vi "test2.vi"() -> ()   [LabVIEW 2024]
panel:
  out "transmission time":dbl
  out "unsigned byte array":u8[](array[numeric])
  out "data out":string
  in  "stop":bool
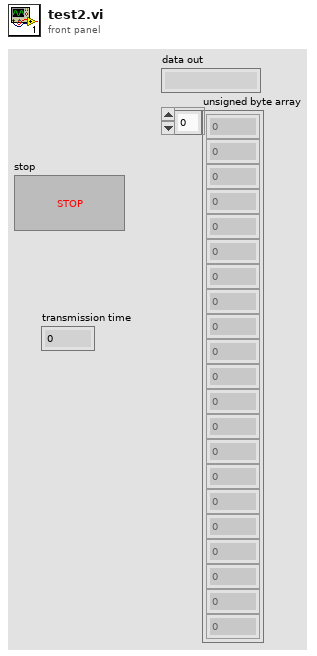
[diagram p1: front panel]
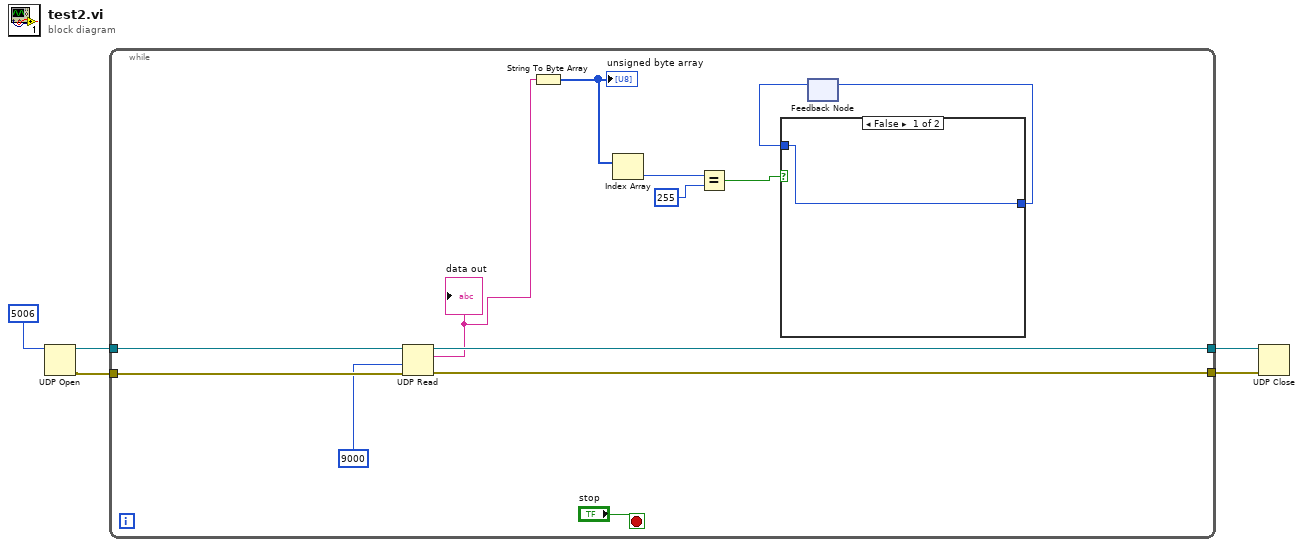
[diagram p0: block diagram]
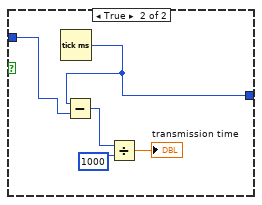
[diagram p2: hidden frame]
diagram:
  n1 = UDP Open(11:u16 5006 ("port")) -> (port=w5:refnum<k16>, 0:w2:errorcluster)  [unwired: 4 in, 1 out]
  n2 = while {
    tunnel: w5 -> [w17]
    tunnel: [w16] -> w4
    tunnel: [w15] -> w3
    tunnel: w2 -> [w14]
    stop <- "stop" stop-if-true
    n3 = UDP Read(connection ID=w17, timeout ms (25000)=9000, 8:w14) -> (data out=w6:string, error out=w15:errorcluster, 3:w16:refnum<k16>)  [unwired: 1 in, 2 out]
    "data out" <- w6
    n4 = String To Byte Array(string=w6) -> (unsigned byte array=w9:u8[])
    "unsigned byte array" <- w9
    n5 = Index Array(array=w9) -> (element=w10:u8)  [unwired: 1 in]
    n6 = Equal?(x=w10, y=u8 255) -> (x = y?=w12:bool)
    n7 = feedback #1() -> (w11:u32)  [unwired: 1 in]
    n8 = case shown="False" w12 {
      tunnel: [w19 w24] -> w7
      tunnel: w11 -> [w19 w23]
      frame False {
      }
      frame True {
        n9 = Tick Count (ms)() -> (millisecond timer value=w24:u32)
        n10 = Subtract(x=w24, y=w23) -> (x-y=w22:u32)
        n11 = Divide(x=w22, y=u32 1000) -> (x/y=→"transmission time":dbl)
      }
    }
    n12 = feedback-in #1(w7) -> ()
  }
  n13 = UDP Close(connection ID=w4, 8:w3) -> ()  [unwired: 2 out]
